vi "writeVideoConfigFile.vi"() -> ()   [LabVIEW 2019]
uses:
  AimingBeamVideoConfig.ctl
  <vilib>/Utility/config.llb/Write Key (I32).vi
  <vilib>/Utility/config.llb/Write Key (Boolean).vi
  <vilib>/Utility/config.llb/Write Key (Double).vi
  <vilib>/Utility/config.llb/NI_LVConfig.lvlib
panel:
  out "error out":errorcluster
  in  "error in (no error)":errorcluster
  in  "Aiming Beam Config":T1={"DeCon Channel"=enum."1", "Scale Bar"=FALSE, "Scale Low"=3.0, "Scale High"=8.0, "ANSI"=20.0, "Radius"=1.0, "3D?"=FALSE, "Firefly?"=FALSE, "Pentero?"=FALSE}
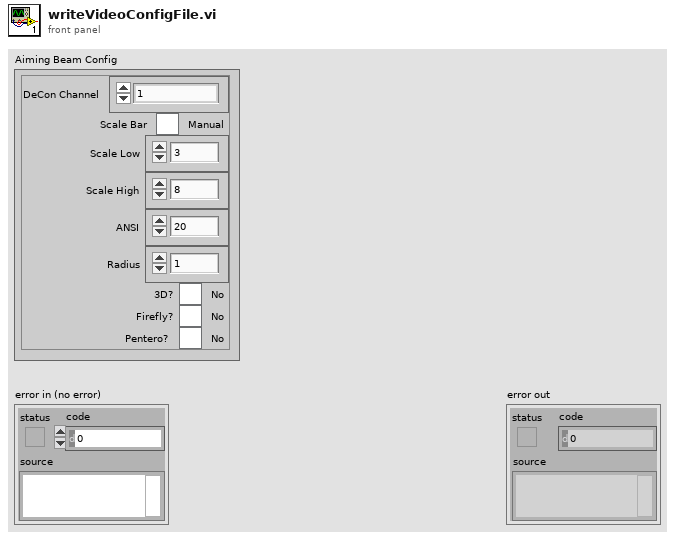
[diagram p1: front panel]
types:
  T1 = typedef "AimingBeamVideoConfig.ctl" = cluster{"DeCon Channel":enum16{"1", "2", "3"}, "Scale Bar":bool, "Scale Low":dbl, "Scale High":dbl, "ANSI":dbl, "Radius":dbl, "3D?":bool, "Firefly?":bool, "Pentero?":bool}
  T2 = typedef "NI_LVConfig.lvlib/Config Data RefNum.ctl" = refnum<k1>
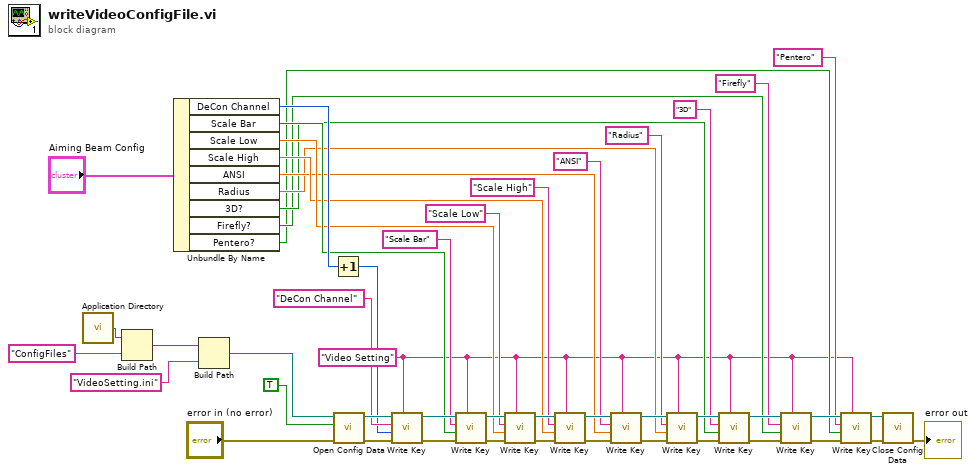
[diagram p0: block diagram]
diagram:
  w1 = "Video Setting" ("section")
  n1 = call <vilib>:"Application Directory.vi"() -> ("Application Directory"=w47:path)
  n2 = Build Path(base path=w47, name or relative path="ConfigFiles") -> (appended path=w45:path)
  n3 = Unbundle By Name("Aiming Beam Config") -> ("DeCon Channel"=w39:enum16{"1", "2", "3"}, "Scale Bar"=w33:bool, "Scale Low"=w29:dbl, "Scale High"=w26:dbl, "ANSI"=w21:dbl, "Radius"=w17:dbl, "3D?"=w13:bool, "Firefly?"=w9:bool, "Pentero?"=w5:bool)
  n4 = Build Path(base path=w45, name or relative path="VideoSetting.ini") -> (appended path=w43:path)
  n5 = Increment(x=w39) -> (x+1=w38:enum16{"1", "2", "3"})
  n6 = call <vilib>:"Open Config Data.vi"("error in (no error)"="error in (no error)", "create file if necessary (T)"=TRUE, "configuration file path"=w43) -> ("error out"=w37:errorcluster, "refnum"=w42:T2)  [unwired: 6 in, 1 out]
  n7 = call-poly <vilib>:"Write Key.vi"("section"=w1, "error in (no error)"=w37, "value"=w38, "key"="DeCon Channel", "refnum"=w42) -> ("error out"=w35:errorcluster, "refnum out"=w36:T2)  [unwired: 4 in, 1 out]
  n8 = call-poly <vilib>:"Write Key.vi"("section"=w1, "error in (no error)"=w35, "value"=w33, "key"="Scale Bar", "refnum"=w36) -> ("error out"=w31:errorcluster, "refnum out"=w32:T2)  [unwired: 4 in, 1 out]
  n9 = call-poly <vilib>:"Write Key.vi"("section"=w1, "error in (no error)"=w31, "value"=w29, "key"="Scale Low", "refnum"=w32) -> ("error out"=w25:errorcluster, "refnum out"=w28:T2)  [unwired: 4 in, 1 out]
  n10 = call-poly <vilib>:"Write Key.vi"("section"=w1, "error in (no error)"=w25, "value"=w26, "key"="Scale High", "refnum"=w28) -> ("error out"=w23:errorcluster, "refnum out"=w24:T2)  [unwired: 4 in, 1 out]
  n11 = call-poly <vilib>:"Write Key.vi"("section"=w1, "error in (no error)"=w23, "value"=w21, "key"="ANSI", "refnum"=w24) -> ("error out"=w19:errorcluster, "refnum out"=w20:T2)  [unwired: 4 in, 1 out]
  n12 = call-poly <vilib>:"Write Key.vi"("section"=w1, "error in (no error)"=w19, "value"=w17, "key"="Radius", "refnum"=w20) -> ("error out"=w15:errorcluster, "refnum out"=w16:T2)  [unwired: 4 in, 1 out]
  n13 = call-poly <vilib>:"Write Key.vi"("section"=w1, "error in (no error)"=w15, "value"=w13, "key"="3D", "refnum"=w16) -> ("error out"=w11:errorcluster, "refnum out"=w12:T2)  [unwired: 4 in, 1 out]
  n14 = call-poly <vilib>:"Write Key.vi"("section"=w1, "error in (no error)"=w11, "value"=w9, "key"="Firefly", "refnum"=w12) -> ("error out"=w7:errorcluster, "refnum out"=w8:T2)  [unwired: 4 in, 1 out]
  n15 = call-poly <vilib>:"Write Key.vi"("section"=w1, "error in (no error)"=w7, "value"=w5, "key"="Pentero", "refnum"=w8) -> ("error out"=w3:errorcluster, "refnum out"=w4:T2)  [unwired: 4 in, 1 out]
  n16 = call <vilib>:"Close Config Data.vi"("error in (no error)"=w3, "refnum"=w4) -> ("error out"=→"error out":errorcluster)  [unwired: 8 in, 1 out]
